vi "Configure Device.vi"(8 "error in (no error)":errorcluster, 10 "Max beams":dbl, 11 "WS1021 in":refnum<class "WS1021.lvclass">) -> (0 "error out":errorcluster, 3 "WS1021 out":refnum<class "WS1021.lvclass">)   [LabVIEW 2020, in "WS1021.lvclass"]
doc: "Interface for configuring the device for testing"
uses:
  WS1021.lvclass
  Toggle 8.lvclass
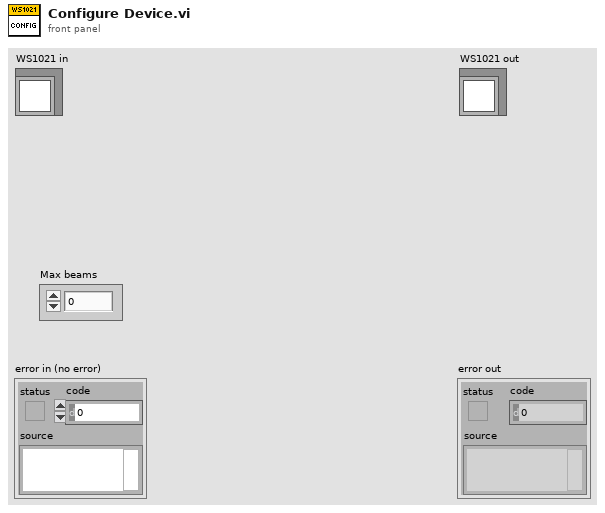
[diagram p1: front panel]
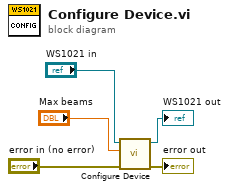
[diagram p0: block diagram]
diagram:
  n1 = call-parent "Configure Device.vi"("error in (no error)"="error in (no error)", "Max beams"="Max beams", "Toggle 8 in"="WS1021 in") -> ("error out"=→"error out":errorcluster, "Toggle 8 out"=→"WS1021 out":refnum<class "WS1021.lvclass">)  [unwired: 7 in]
